vi "Get Datatype Information.vi"(8 "error in (no error)":errorcluster, 10 "Type Name":string, 11 "TwinCAT ADS in":refnum<class "TwinCAT ADS.lvclass">) -> (0 "error out":errorcluster, 1 ".NET AdsDataType":refnum<k24>, 3 "TwinCAT ADS out":refnum<class "TwinCAT ADS.lvclass">)   [LabVIEW 2018, in "TwinCAT ADS.lvclass"]
uses:
  TwinCAT ADS.lvclass
  TwinCAT.Ads
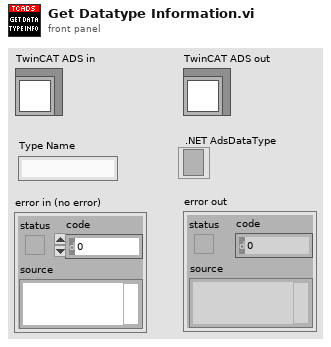
[diagram p1: front panel]
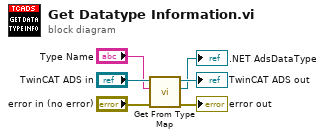
[diagram p0: block diagram]
diagram:
  n1 = call "Get From Type Map.vi"("error in (no error)"="error in (no error)", "Type Name"="Type Name", "TwinCAT ADS in"="TwinCAT ADS in") -> ("error out"=→"error out":errorcluster, ".NET AdsDataType"=→".NET AdsDataType":refnum<k24>, "TwinCAT ADS out"=→"TwinCAT ADS out":refnum<class "TwinCAT ADS.lvclass">)  [unwired: 6 in]
